vi "punto #3.vi"() -> ()   [LabVIEW 2017]
panel:
  out "tem. min":bool
  out "tem.max":bool
  out "decremento":bool
  out "incremento":bool
  in  "temp. min":dbl
  in  "temp. max":dbl
  in  "selector":bool
  in  "incremento":dbl(knob) scale=0.0..10.0
  in  "decremento":dbl(knob) scale=0.0..10.0
  in  "rata(5°c/seg)":dbl(knob) scale=0.0..10.0
  out "sensor de temperatura":dbl(slide) scale=0.0..100.0
  # "incremento"
  # "decremento"
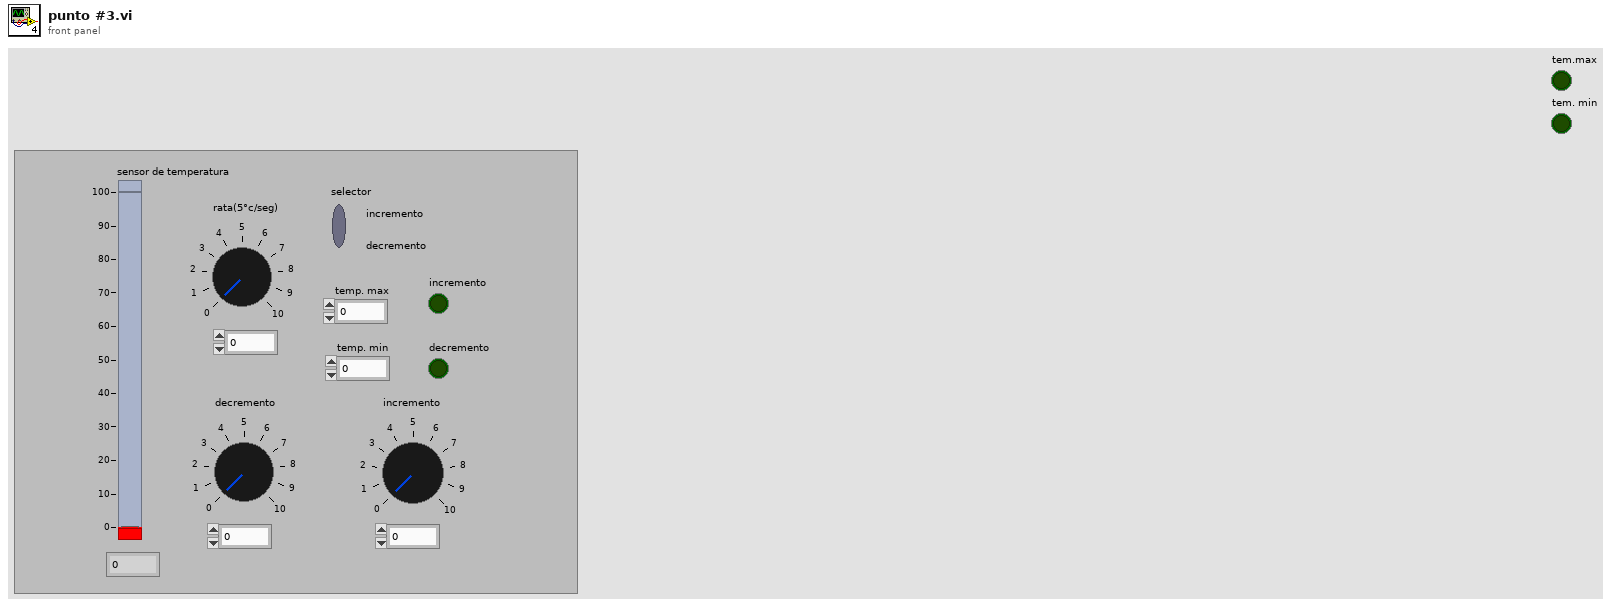
[diagram p1: front panel]
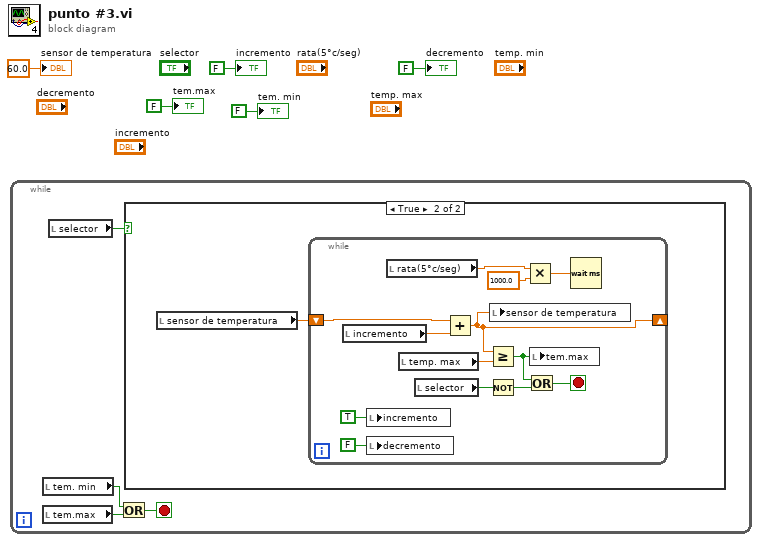
[diagram p0: block diagram]
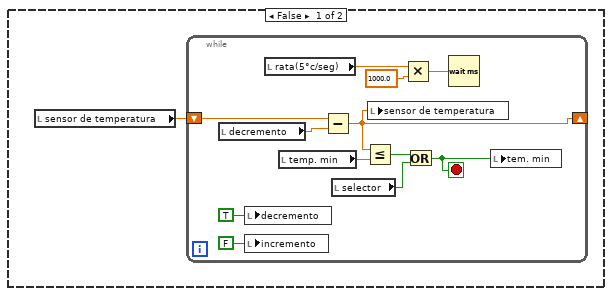
[diagram p2: hidden frame]
diagram:
  n1 = while {
    stop <- w6 stop-if-true
    n2 = local read "tem. min"() -> (w8:bool)
    n3 = local read "tem.max"() -> (w7:bool)
    n4 = local read "selector"() -> (w9:bool)
    n5 = Or(x=w8, y=w7) -> (x .or. y?=w6:bool)
    n6 = case shown="True" w9 {
      frame False {
        n7 = local read "sensor de temperatura"() -> (w10:dbl)
        n8 = while {
          shift-right: [w21] -> _
          shift-left: w10 -> [w22]
          stop <- w11 stop-if-true
          n9 = local read "decremento"() -> (w20:dbl)
          n10 = local write "decremento"(TRUE ("decremento")) -> ()
          n11 = local write "incremento"(FALSE ("incremento")) -> ()
          n12 = local read "rata(5°c/seg)"() -> (w17:dbl)
          n13 = local read "temp. min"() -> (w19:dbl)
          n14 = Subtract(x=w22, y=w20) -> (x-y=w21:dbl)
          n15 = local read "selector"() -> (w12:bool)
          n16 = Less Or Equal?(x=w21, y=w19) -> (x <= y?=w13:bool)
          n17 = local write "sensor de temperatura"(w21) -> ()
          n18 = Multiply(x=w17, y=1000.0) -> (x*y=w18:dbl)
          n19 = Or(x=w13, y=w12) -> (x .or. y?=w11:bool)
          n20 = Wait (ms)(milliseconds to wait=w18) -> ()  [unwired: 1 out]
          n21 = local write "tem. min"(w11) -> ()
        }
      }
      frame True {
        n22 = local read "sensor de temperatura"() -> (w23:dbl)
        n23 = while {
          shift-right: [w34] -> _
          shift-left: w23 -> [w36]
          stop <- w28 stop-if-true
          n24 = local read "incremento"() -> (w35:dbl)
          n25 = local write "incremento"(TRUE ("incremento")) -> ()
          n26 = local write "decremento"(FALSE ("decremento")) -> ()
          n27 = local read "rata(5°c/seg)"() -> (w31:dbl)
          n28 = local read "temp. max"() -> (w33:dbl)
          n29 = local read "selector"() -> (w29:bool)
          n30 = Add(x=w36, y=w35) -> (x+y=w34:dbl)
          n31 = Greater Or Equal?(x=w34, y=w33) -> (x >= y?=w27:bool)
          n32 = Not(x=w29) -> (.not. x?=w26:bool)
          n33 = local write "sensor de temperatura"(w34) -> ()
          n34 = Multiply(x=w31, y=1000.0) -> (x*y=w32:dbl)
          n35 = Or(x=w27, y=w26) -> (x .or. y?=w28:bool)
          n36 = local write "tem.max"(w27) -> ()
          n37 = Wait (ms)(milliseconds to wait=w32) -> ()  [unwired: 1 out]
        }
      }
    }
  }
  "sensor de temperatura" <- 60.0 ("sensor de temperatura")
  "incremento" <- FALSE ("incremento")
  "decremento" <- FALSE ("decremento")
  "tem.max" <- FALSE ("tem.max")
  "tem. min" <- FALSE ("tem. min")
